vi "Write Sender.vi"(10 "Sender":refnum<class "Sender.lvclass">, 11 "Go To Destroy Msg in":refnum<class "Go To Destroy Msg.lvclass">) -> (3 "Go To Destroy Msg out":refnum<class "Go To Destroy Msg.lvclass">)   [LabVIEW 2020, in "jettl.lvlib" / "Go To Destroy Msg.lvlib" / "Go To Destroy Msg.lvclass"]
uses:
  Go To Destroy Msg.lvclass
  Sender/Sender/Sender.lvclass
  Go To Destroy Msg.lvclass/Go To Destroy Msg.ctl
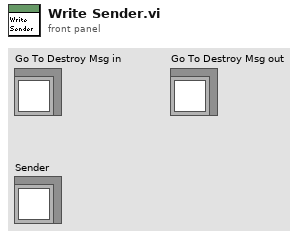
[diagram p1: front panel]
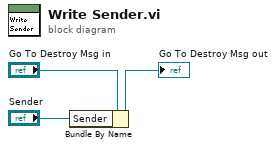
[diagram p0: block diagram]
diagram:
  n1 = Bundle By Name(cluster="Go To Destroy Msg in", "Sender"="Sender") -> (→"Go To Destroy Msg out":refnum<class "Go To Destroy Msg.lvclass">)
